vi "change working directory.vi"(10 "Application Name":string="LJstream", 11 "Working Directory In":path) -> (3 "Working Directory Out":path)   [LabVIEW 2021]
uses:
  <vilib>/registry/registry.llb/Registry RtKey.ctl
  <vilib>/registry/registry.llb/Write Registry Value Simple STR.vi
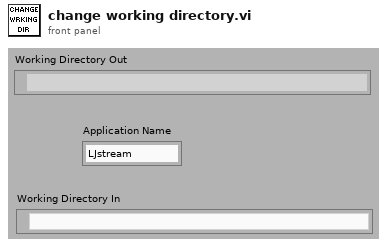
[diagram p1: front panel]
types:
  T1 = enum16{"open", "open or create", "create or replace", "create", "open (read only)"}
  T2 = typedef "Registry RtKey.ctl" = enum32{"HKEY_CLASSES_ROOT", "HKEY_CURRENT_USER", "HKEY_LOCAL_MACHINE", "HKEY_USERS", "HKEY_PERFORMANCE_DATA", "HKEY_CURRENT_CONFIG", "HKEY_DYN_DATA"}
  T3 = enum32{"existing file", "new file", "new or existing file", "existing dir", "new dir", "new or existing dir", "existing file (use LLBs)", "new file (use LLBs)", "new or existing file (use LLBs)", "new or existing file or directory (use LLBs)"}
  T4 = typedef "Registry refnum.ctl" = refnum<k1>
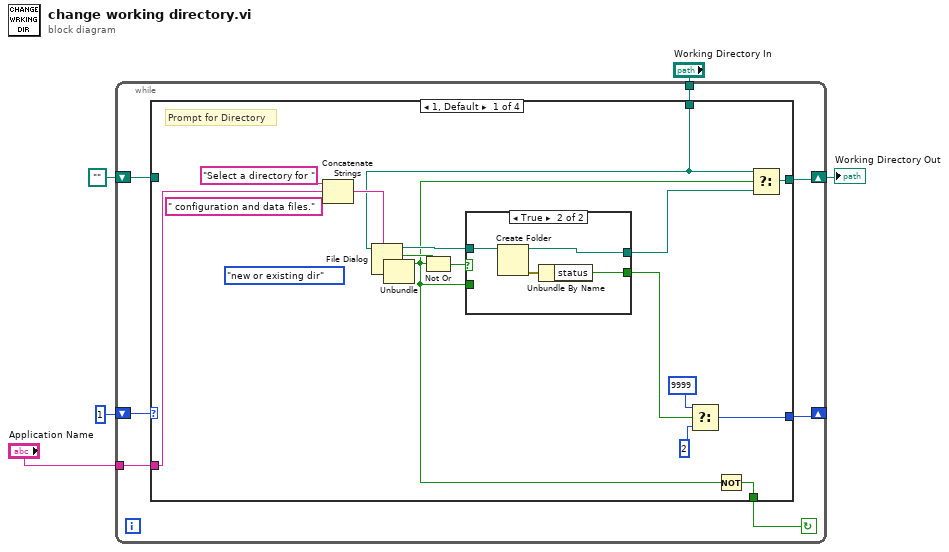
[diagram p0: block diagram]
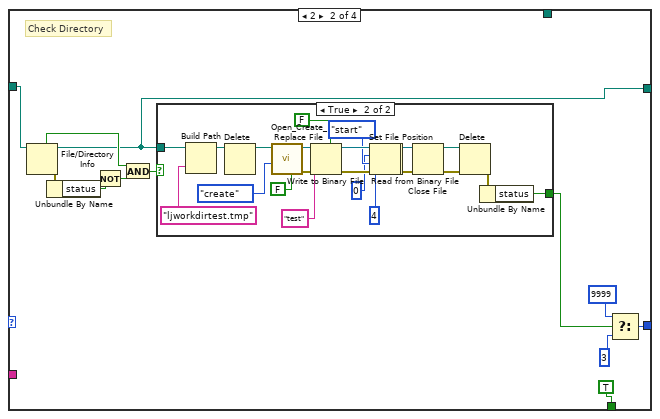
[diagram p3: hidden frame]
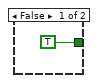
[diagram p4: hidden frame]
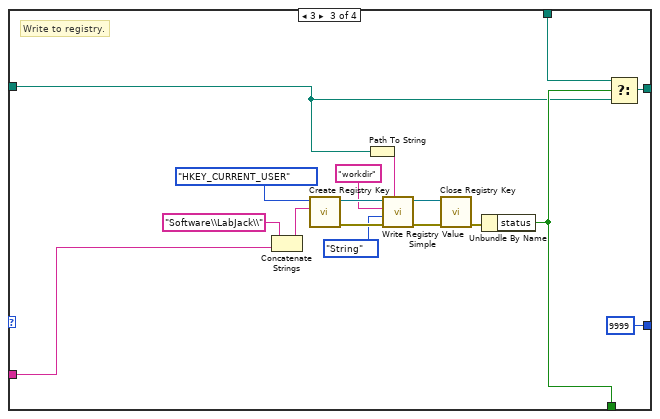
[diagram p5: hidden frame]
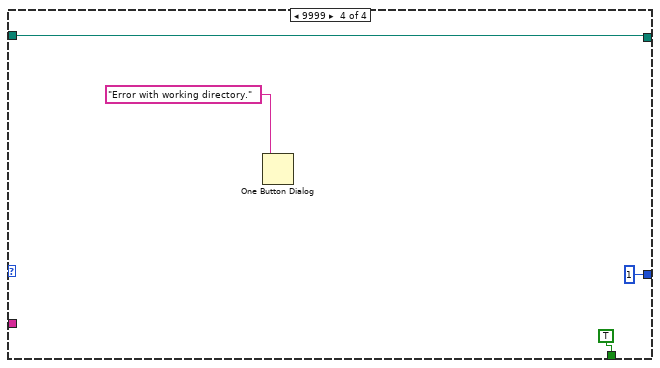
[diagram p6: hidden frame]
diagram:
  n1 = while {
    tunnel: "Working Directory In" -> [w6]
    tunnel: "Application Name" -> [w7]
    shift-left: path "" -> [w8]
    shift-right: [w10] -> w3
    shift-left: 1 -> [w12]
    shift-right: [w11] -> _
    stop <- w9 continue-if-true
    n2 = case shown="1, Default" w12 {
      tunnel: [w26 w39 9999 ("t") 1 ("t")] -> w11
      tunnel: [w17 w36 w75 w89] -> w10
      tunnel: [w19 TRUE ("status") w74 TRUE ("status")] -> w9
      tunnel: w8 -> [_ w47 w72 w89]
      tunnel: w7 -> [w20 _ w77 _]
      tunnel: w6 -> [w14 _ w73 _]
      frame 1, Default {
        (unwired) T3."new or existing dir" ("select mode (2)")
        # "Prompt for Directory"
        n3 = Concatenate Strings("Select a directory for " ("Substring"), w20, " configuration and data files." ("Substring")) -> (w21:string)
        n4 = File Dialog(7:w21, 11:w14) -> (0:w13:errorcluster, 1:w16:bool, 2:w28:bool, 3:w29:path)  [unwired: 5 in]
        n5 = Unbundle(w13) -> ()  [unwired: 3 out]
        n6 = Not Or(1:w16, 2:w28) -> (0:w27:bool)
        n7 = case shown="True" w27 {
          tunnel: w29 -> [w30 w35]
          tunnel: [w30 w33] -> w15
          tunnel: [w31 w32] -> w18
          tunnel: w16 -> [w31 _]
          frame False {
          }
          frame True {
            n8 = Create Folder(path (use dialog)=w35) -> (created path=w33:path, error out=w34:errorcluster)  [unwired: 2 in, 1 out]
            n9 = Unbundle By Name(w34) -> ("status"=w32:bool)
          }
        }
        n10 = Select(t=9999, s=w18, f=2) -> (s? t:f=w26:i32)
        n11 = Not(x=w16) -> (.not. x?=w19:bool)
        n12 = Select(t=w14, s=w16, f=w15) -> (s? t:f=w17:path)
      }
      frame 2 {
        # "Check Directory"
        n13 = File/Directory Info(path=w47) -> (path out=w36:path, directory=w43:bool, error out=w46:errorcluster)  [unwired: 1 in, 4 out]
        n14 = Unbundle By Name(w46) -> ("status"=w45:bool)
        n15 = Not(x=w45) -> (.not. x?=w44:bool)
        n16 = And(x=w43, y=w44) -> (x .and. y?=w42:bool)
        n17 = case shown="True" w42 {
          tunnel: w36 -> [_ w64]
          tunnel: [TRUE ("status") w56] -> w37
          frame False {
          }
          frame True {
            n18 = Build Path(base path=w64, name or relative path="ljworkdirtest.tmp") -> (appended path=w62:path)
            n19 = Delete(path (use dialog)=w62) -> (deleted path=w71:path)  [unwired: 4 in, 2 out]
            n20 = call <vilib>:"Open_Create_Replace File.vi"("advisory dialog? (display:T)"=FALSE, "function (open:0)"=T1."create", "file path"=w71) -> ("error out"=w67:errorcluster, "refnum"=w70:refnum<file>)  [unwired: 5 in, 2 out]
            n21 = Write to Binary File(file (use dialog)=w70, data="test", error in=w67, 5:FALSE ("prepend array or string size? (T)")) -> (refnum out=w69:refnum<file>, error out=w66:errorcluster)  [unwired: 2 in, 1 out]
            n22 = Set File Position(offset (in bytes) (0)=0 ("pos offset (0)"), refnum=w69, from (0:start)=enum16{"start", "end", "current"}."start" ("pos mode (0:2)"), error in=w66) -> (refnum out=w50:refnum<file>, error out=w49:errorcluster)
            n23 = Read from Binary File(8:w49, 10:4 ("count"), 11:w50) -> (0:w65:errorcluster, 3:w68:refnum<file>)  [unwired: 3 in, 2 out]
            n24 = Close File(refnum=w68, error in=w65) -> (path=w59:path, error out=w58:errorcluster)
            n25 = Delete(path (use dialog)=w59, error in=w58) -> (error out=w57:errorcluster)  [unwired: 3 in, 2 out]
            n26 = Unbundle By Name(w57) -> ("status"=w56:bool)
          }
        }
        n27 = Select(t=9999, s=w37, f=3) -> (s? t:f=w39:i32)
      }
      frame 3 {
        # "Write to registry."
        n28 = Concatenate Strings("Software\\LabJack\\" ("subkey"), w77) -> (w78:string)
        n29 = call <vilib>:"Create Registry Key.vi"("subkey"=w78, "root key (HKEY_LOCAL_MACHINE)"=Registry_RtKey."HKEY_CURRENT_USER") -> ("error out"=w86:errorcluster, "refnum out"=w85:T4)  [unwired: 7 in, 1 out]
        n30 = Path To String(path=w72) -> (string=w80:string)
        n31 = call-poly <vilib>:"Write Registry Value Simple.vi"("String/Binary data"=w80, "error in (no error)"=w86, "simple data type"=enum16{"String", "Binary", "DWORD"}."String", "value"="workdir", "refnum"=w85) -> ("error out"=w83:errorcluster, "refnum out"=w84:T4)  [unwired: 3 in]
        n32 = call <vilib>:"Close Registry Key.vi"("error in (no error)"=w83, "refnum"=w84) -> ("error out"=w76:errorcluster)  [unwired: 5 in]
        n33 = Unbundle By Name(w76) -> ("status"=w74:bool)
        n34 = Select(t=w73, s=w74, f=w72) -> (s? t:f=w75:path)
      }
      frame 9999 {
        n35 = One Button Dialog(message="Error with working directory.") -> ()  [unwired: 1 in, 1 out]
      }
    }
  }
  "Working Directory Out" <- w3
